vi "GE 5565PIORC.Registers.RFM Control and Status.Read (U32).vi"(7 "Mask (0xFFFFFFFF)":u32=4294967295 format="%.0x", 8 "error in (no error)":errorcluster, 10 "Register":T1=8 items=["BRV"=0, "BID"=1, "BRB"=2, "NID"=4, "LCSR1"=8, "LISR"=16, "LIER"=20, "NTD"=24, "NTN"=28, "NIC"=29, "ISD1"=32, "SID1"=36, "ISD2"=40, "SID2"=44, "ISD3"=48, "SID3"=52, "ISD4"=56, "SID4"=60], 11 "GE 5565PIORC in":refnum<class "GE 5565PIORC.lvclass">) -> (0 "error out":errorcluster, 1 "Value":u32, 3 "GE 5565PIORC out":refnum<class "GE 5565PIORC.lvclass">)   [LabVIEW 2017, in "GE 5565PIORC.lvclass"]
uses:
  GE 5565PIORC.lvclass
  GE 5565PIORC.Registers.RFM Control and Status.ctl
  <vilib>/Instr/_visa.llb/VISA Register Access Address Space.ctl
  GE 5565PIORC.lvclass/GE 5565PIORC.ctl
  Methods/GE 5565PIORC.Registers.Read (U32).vi
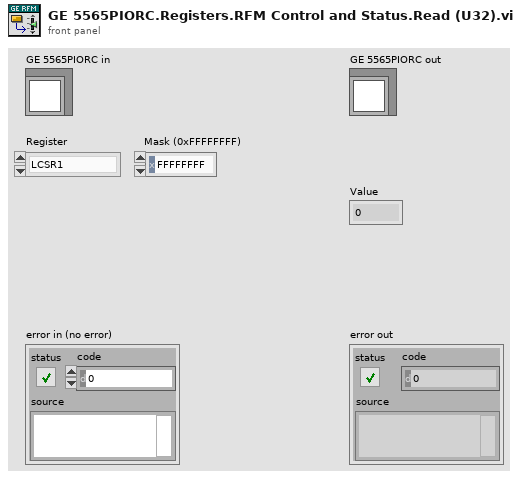
[diagram p1: front panel]
types:
  T1 = typedef "GE 5565PIORC.lvclass/GE 5565PIORC.Registers.RFM Control and Status.ctl" = u32
  T2 = typedef "VISA Register Access Address Space.ctl" = u16
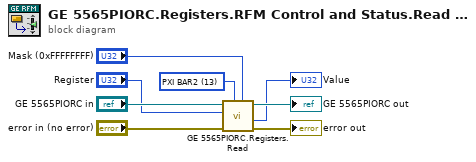
[diagram p0: block diagram]
diagram:
  w5 = T2 13 items=["VXI/VME A16"=1, "VXI/VME A24"=2, "VXI/VME A32"=3, "VXI/VME A64"=4, "PXI Memory Allocations"=9, "PXI Configuration"=10, "PXI BAR0"=11, "PXI BAR1"=12, "PXI BAR2"=13, "PXI BAR3"=14, "PXI BAR4"=15, "PXI BAR5"=16] ("Address Space")
  n1 = call-poly "GE 5565PIORC.Registers.Read.vi"("Mask (0xFFFFFFFF)"="Mask (0xFFFFFFFF)", "Address Space"=w5, "error in (no error)"="error in (no error)", "Offset"="Register", "GE 5565PIORC in"="GE 5565PIORC in") -> ("error out"=→"error out":errorcluster, "Value"=→"Value":u32, "GE 5565PIORC out"=→"GE 5565PIORC out":refnum<class "GE 5565PIORC.lvclass">)  [unwired: 4 in]
